vi "SwerveOdometry_Execute.vi"(6 "Initial Pose":T1={"TRANSLATION"={"X"=0.0, "Y"=0.0}, "ROTATION"={"VALUE"=0.0, "COS"=1.0, "SIN"=0.0}} {"ROTATION"."SIN" format="%13.4f"; "ROTATION"."COS" format="%13.4f"; "ROTATION"."VALUE" format="%13.4f"; "TRANSLATION"."Y" format="%14.3f"; "TRANSLATION"."X" format="%14.3f"}, 8 "Init":bool, 9 "Rotation":T3={"VALUE"=0.0, "COS"=1.0, "SIN"=0.0} {"SIN" format="%13.4f"; "COS" format="%13.4f"; "VALUE" format="%13.4f"}, 10 "Swerve Module Positions":T4[](array[typedef]) {"Angle"."SIN" format="%13.4f"; "Angle"."COS" format="%13.4f"; "Angle"."VALUE" format="%13.4f"}, 11 "SWERVE_DRIVE_KINEMATICS":T5 {"SavedModuleStates"."Angle"."SIN" format="%13.4f"; "SavedModuleStates"."Angle"."COS" format="%13.4f"; "SavedModuleStates"."Angle"."VALUE" format="%13.4f"; "PrevCoR"."Y" format="%14.3f"; "PrevCoR"."X" format="%14.3f"; "Modules"."Y" format="%14.3f"; "Modules"."X" format="%14.3f"}) -> (0 "Error":bool, 3 "Current Pose":T1={"TRANSLATION"={"X"=0.0, "Y"=0.0}, "ROTATION"={"VALUE"=0.0, "COS"=1.0, "SIN"=0.0}} {"ROTATION"."SIN" format="%13.4f"; "ROTATION"."COS" format="%13.4f"; "ROTATION"."VALUE" format="%13.4f"; "TRANSLATION"."Y" format="%14.3f"; "TRANSLATION"."X" format="%14.3f"}, 4 "SWERVE_DRIVE_ODOMETRY":T8={"POSE"={"TRANSLATION"={"X"=0.0, "Y"=0.0}, "ROTATION"={"VALUE"=0.0, "COS"=1.0, "SIN"=0.0}}, "GyroOffset"={"VALUE"=0.0, "COS"=1.0, "SIN"=0.0}, "PreviousAngle"={"VALUE"=0.0, "COS"=1.0, "SIN"=0.0}, "PrevModulePositions"=[], "NumModules"=0} {"PrevModulePositions"."Angle"."SIN" format="%13.4f"; "PrevModulePositions"."Angle"."COS" format="%13.4f"; "PrevModulePositions"."Angle"."VALUE" format="%13.4f"; "PreviousAngle"."SIN" format="%13.4f"; "PreviousAngle"."COS" format="%13.4f"; "PreviousAngle"."VALUE" format="%13.4f"; "GyroOffset"."SIN" format="%13.4f"; "GyroOffset"."COS" format="%13.4f"; "GyroOffset"."VALUE" format="%13.4f"; "POSE"."ROTATION"."SIN" format="%13.4f"; "POSE"."ROTATION"."COS" format="%13.4f"; "POSE"."ROTATION"."VALUE" format="%13.4f"; "POSE"."TRANSLATION"."Y" format="%14.3f"; "POSE"."TRANSLATION"."X" format="%14.3f"})   [LabVIEW 2019, in "Trajectory_Library.lvlib"]
doc: "SIngle call LabVIEW function to execute Swerve Drive Odometry to calculate a relative or absolute POSE.\n \nInputs:\n - Swerve_Drive_Kinematics -- cluster -- swerve drive kinematics\n - Swerve Module Positions -- array of cluster -- current module positions.\n - Gyro Value -- rotation2d -- current gyro reading.\n - Init -- boolean -- Reset position to the value of Initial Pose. Odometry is calculated from this position.\n - Initial Pose -- Pose2d -- Pose to use when Init is TRUE. (Optional. Default: 0,0,0 )\n\nReturns\n - Current Pose -- Pose2d -- Current position calculated by Swerve Odometry\n - Error -- boolean -- If TRUE an error has occured\n - Swerve_Drive_Odometry -- cluster -- current value of the swerve drive odometry cluster."
uses:
  Rotation2d_UnaryMinus.vi
  Rotation2d_RotateBy.vi
  Rotation2d_CreateAngle.vi
  Rotation2d_CreateXY.vi
  Util_CalcDist.vi
  Trajectory_Library.lvlib
  TypeDef/TRANSLATION2D.ctl
  TypeDef/ROTATION2D.ctl
  TypeDef/POSE2D.ctl
  TypeDef/SWERVE_DRIVE_ODOMETRY.ctl
  TypeDef/SWERVE_DRIVE_MODULE_POSITION.ctl
  <vilib>/Analysis/Matrix/Datatypes/RealMatrix.ctl
  <vilib>/Analysis/Matrix/NI_Matrix.lvlib
  TypeDef/SWERVE_DRIVE_MODULE_STATE.ctl
  TypeDef/SWERVE_DRIVE_KINEMATICS.ctl
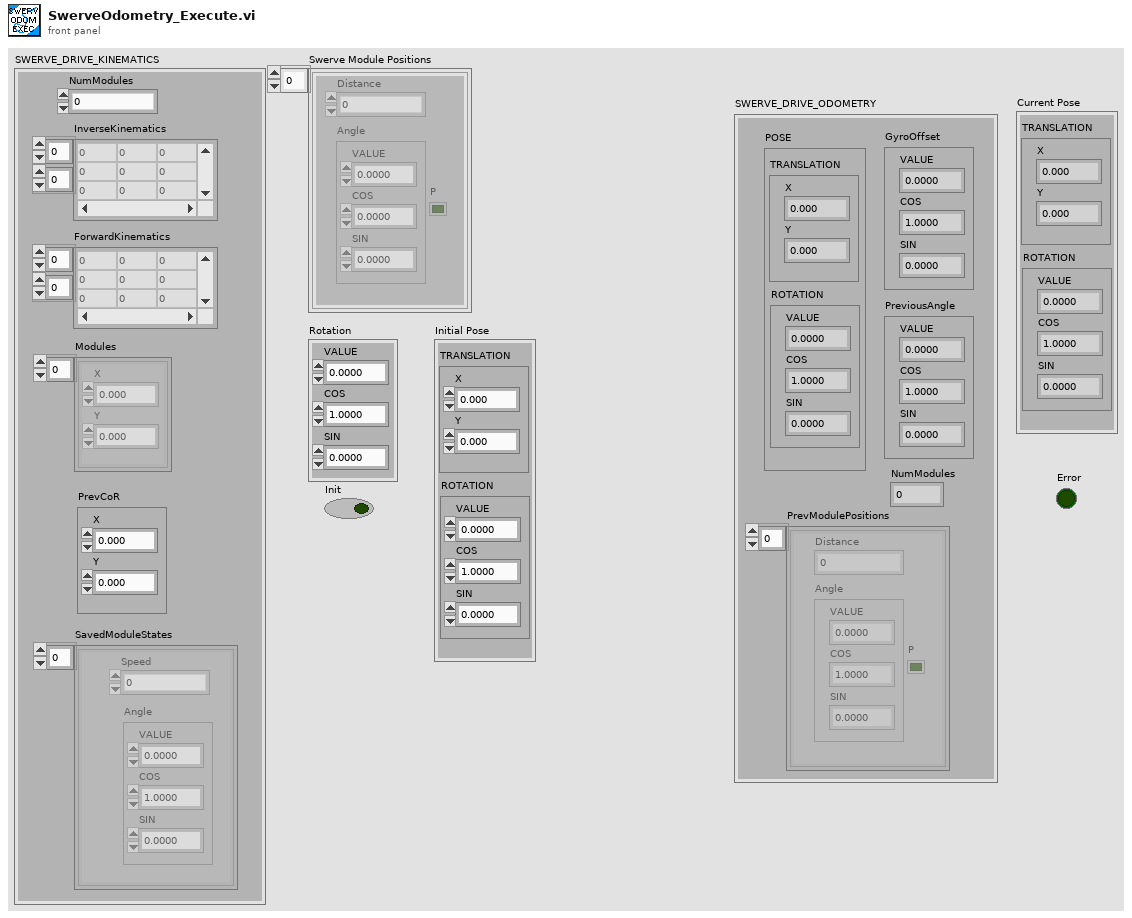
[diagram p1: front panel]
types:
  T1 = typedef "Trajectory_Library.lvlib/POSE2D.ctl" = cluster{"TRANSLATION":T2, "ROTATION":T3}
  T2 = typedef "Trajectory_Library.lvlib/TRANSLATION2D.ctl" = cluster{"X":dbl, "Y":dbl}
  T3 = typedef "Trajectory_Library.lvlib/ROTATION2D.ctl" = cluster{"VALUE":dbl, "COS":dbl, "SIN":dbl}
  T4 = typedef "Trajectory_Library.lvlib/SWERVE_DRIVE_MODULE_POSITION.ctl" = cluster{"Distance":dbl, "Angle":T3, "P":bool}
  T5 = typedef "Trajectory_Library.lvlib/SWERVE_DRIVE_KINEMATICS.ctl" = cluster{"NumModules":i32, "InverseKinematics":T6, "ForwardKinematics":T6, "Modules":T2[], "PrevCoR":T2, "SavedModuleStates":T7[]}
  T6 = typedef "NI_Matrix.lvlib/RealMatrix.ctl" = dbl[][]
  T7 = typedef "Trajectory_Library.lvlib/SWERVE_DRIVE_MODULE_STATE.ctl" = cluster{"Speed":dbl, "Angle":T3}
  T8 = typedef "Trajectory_Library.lvlib/SWERVE_DRIVE_ODOMETRY.ctl" = cluster{"POSE":T1, "GyroOffset":T3, "PreviousAngle":T3, "PrevModulePositions":T4[], "NumModules":i32}
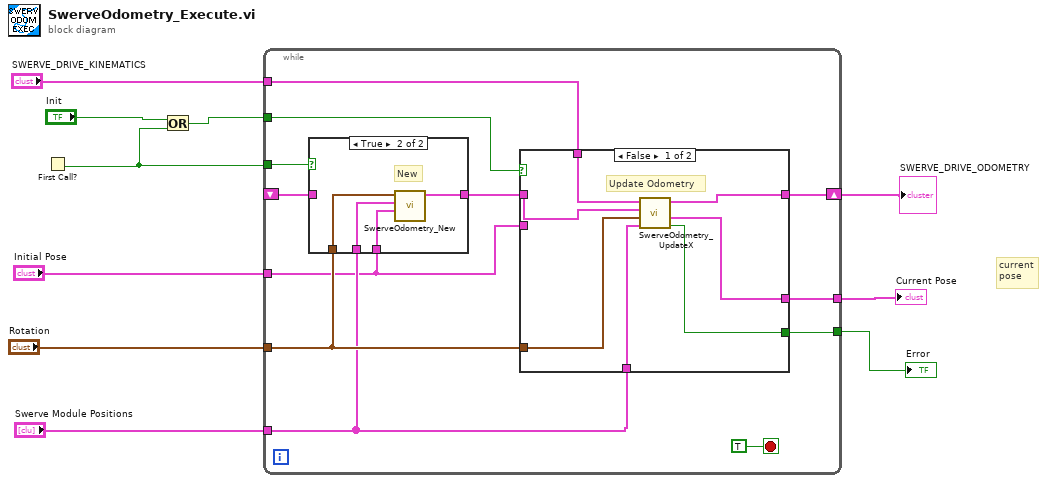
[diagram p0: block diagram]
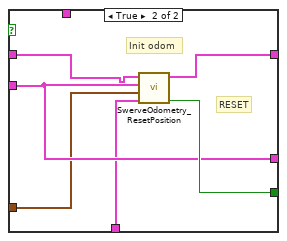
[diagram p3: hidden frame]
diagram:
  # "current\npose"
  n1 = First Call?() -> (First Call?: T/F=w8:bool)
  n2 = Or(x="Init", y=w8) -> (x .or. y?=w9:bool)
  n3 = while {
    tunnel: "Swerve Module Positions" -> [w14]
    tunnel: "Rotation" -> [w15]
    tunnel: "SWERVE_DRIVE_KINEMATICS" -> [w20]
    tunnel: [w18] -> w5
    tunnel: w9 -> [w22]
    shift-right: [w19] -> w6
    shift-left: _ -> [w11]
    tunnel: [w17] -> w7
    tunnel: "Initial Pose" -> [w13]
    tunnel: w8 -> [w16]
    stop <- TRUE stop-if-true
    n4 = case shown="True" w16 {
      tunnel: w15 -> [_ w26]
      tunnel: w14 -> [_ w25]
      tunnel: w13 -> [_ w24]
      tunnel: [w23 w27] -> w12
      tunnel: w11 -> [w23 _]
      frame False {
      }
      frame True {
        # "New"
        n5 = call "SwerveOdometry_New.vi"("InitialPose"=w24, "Module Positions"=w25, "gyroAngle"=w26) -> ("SWERVE_DRIVE_ODOMETRY"=w27:T8)  [unwired: 8 in]
      }
    }
    n6 = case shown="False" w22 {
      tunnel: w12 -> [w29 w38]
      tunnel: w15 -> [w30 w36]
      tunnel: w14 -> [w31 w35]
      tunnel: w20 -> [w28 _]
      tunnel: [w33 w39] -> w19
      tunnel: [w34 w37] -> w18
      tunnel: [w32 w40] -> w17
      tunnel: w13 -> [_ w37]
      frame False {
        # "Update Odometry"
        n7 = call "SwerveOdometry_UpdateX.vi"("module Positions"=w31, "gyroAngle"=w30, "in SWERVE_DRIVE_ODOMETRY"=w29, "SWERVE_DRIVE_KINEMATICS"=w28) -> ("Error"=w32:bool, "robot POSE"=w34:T1, "out SWERVE_DRIVE_ODOMETRY"=w33:T8)  [unwired: 5 in]
      }
      frame True {
        # "RESET"
        # "Init odom"
        n8 = call "SwerveOdometry_ResetPosition.vi"("Module Positions"=w35, "gyroAngle"=w36, "Pose"=w37, "in SWERVE_DRIVE_ODOMETRY"=w38) -> ("Error"=w40:bool, "out SWERVE_DRIVE_ODOMETRY"=w39:T8)  [unwired: 6 in]
      }
    }
  }
  "SWERVE_DRIVE_ODOMETRY" <- w6
  "Error" <- w7
  "Current Pose" <- w5
